vi "Path_Decider.vi"(7 "Second":T3=enum."5", 8 "First":T3=enum."7", 9 "Starting Position":T1) -> (0 "Complete Path Valid?":bool, 1 "Score Second HP Leg":T2={"First Path"="BLANK", "Second Path Needed?"=FALSE, "Second Path"="BLANK"}, 2 "Retrieve Second HP Leg":T2={"First Path"="BLANK", "Second Path Needed?"=FALSE, "Second Path"="BLANK"}, 3 "Score First HP Leg":T2={"First Path"="BLANK", "Second Path Needed?"=FALSE, "Second Path"="BLANK"})   [LabVIEW 2018]
uses:
  Path_Decider.ctl
  pathLeg.ctl
  StartingPosition.ctl
panel:
  in  "Starting Left?":bool
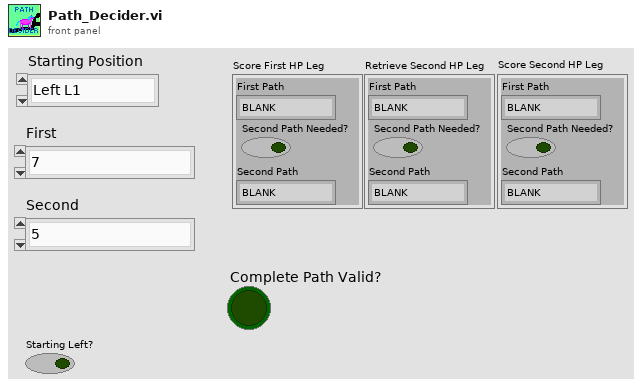
[diagram p1: front panel]
types:
  T1 = typedef "StartingPosition.ctl" = enum16{"Left L1 ", "Middle L1", "Right L1", "Left L2", "Right L2", "Don't Move"}
  T2 = typedef "pathLeg.ctl" = cluster{"First Path":string, "Second Path Needed?":bool, "Second Path":string}
  T3 = typedef "Path_Decider.ctl" = enum16{"1", "2", "3", "4", "5", "6", "7", "8", "Left_Rocket_Front", "Left_Rocket_Rear", "Right_Rocket_Front", "Right_Rocket_Rear"}
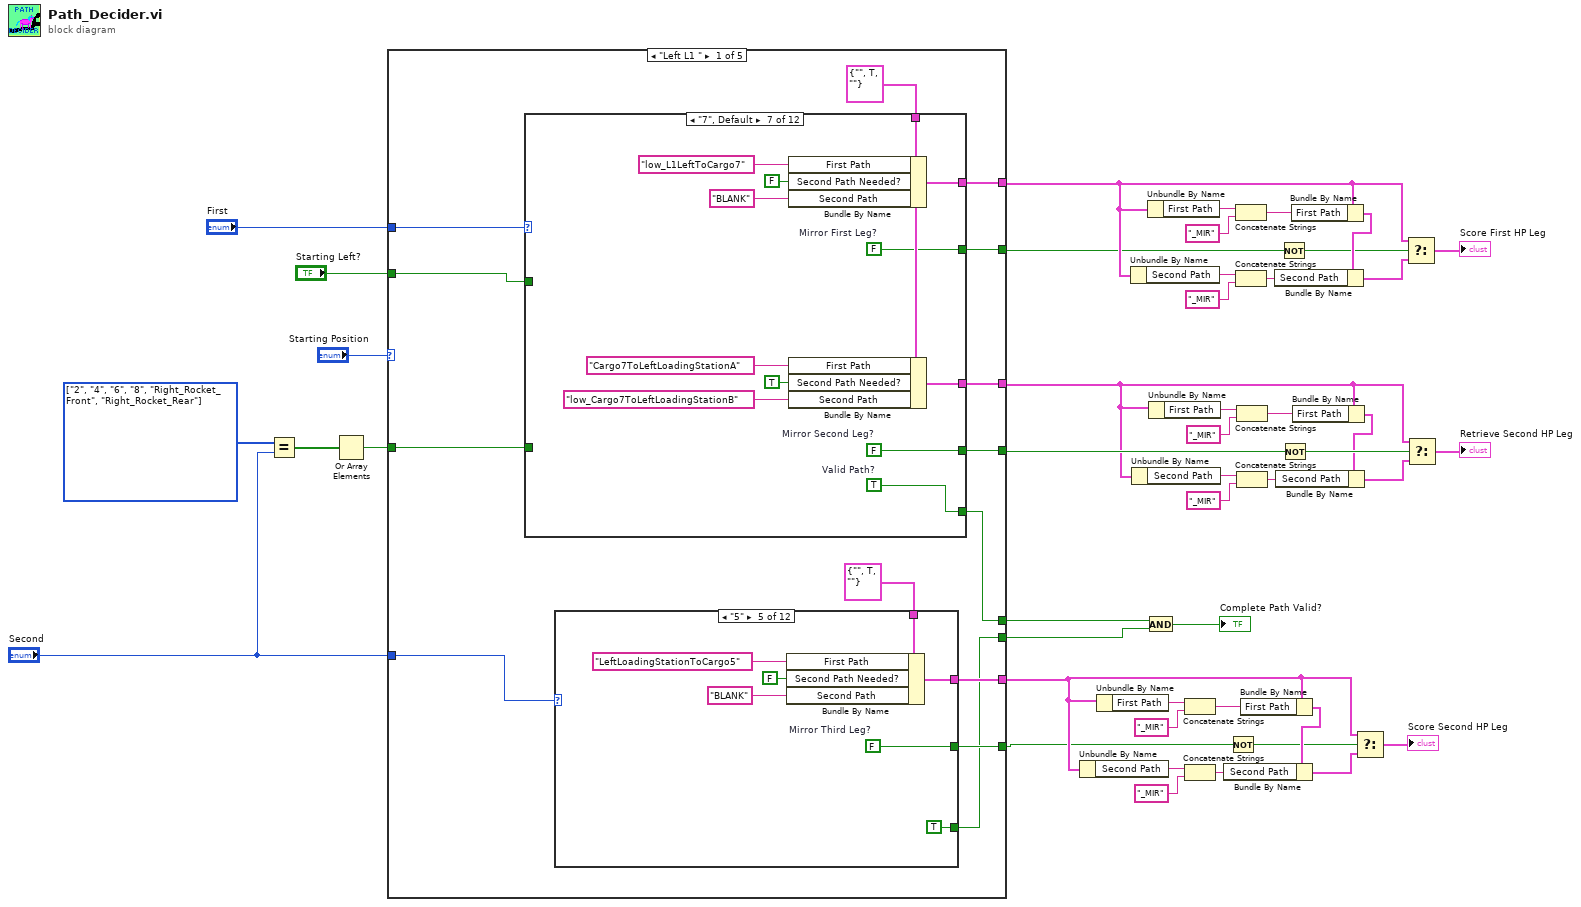
[diagram p0: block diagram]
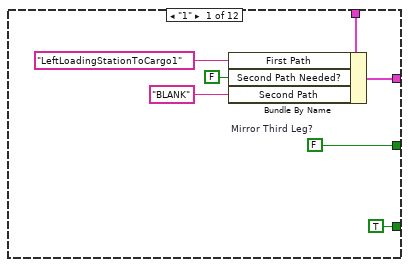
[diagram p2: hidden frame]
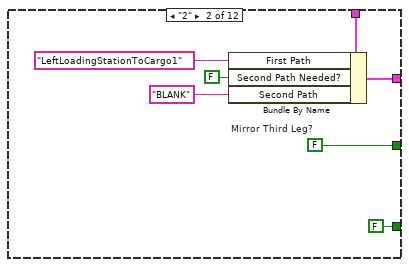
[diagram p3: hidden frame]
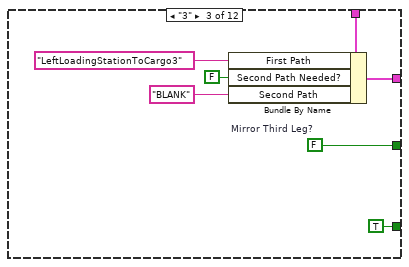
[diagram p4: hidden frame]
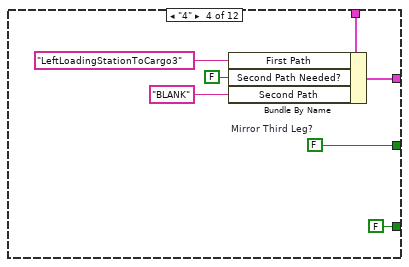
[diagram p5: hidden frame]
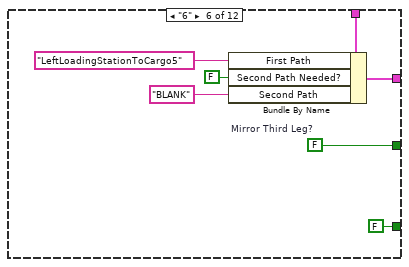
[diagram p6: hidden frame]
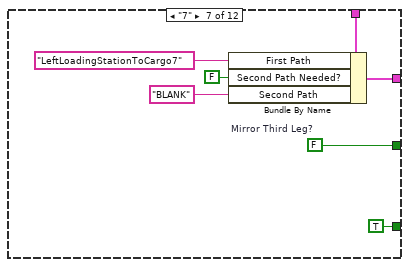
[diagram p7: hidden frame]
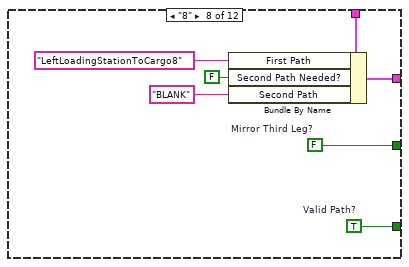
[diagram p8: hidden frame]
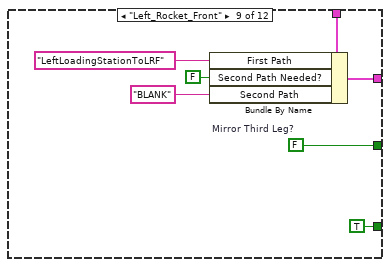
[diagram p9: hidden frame]
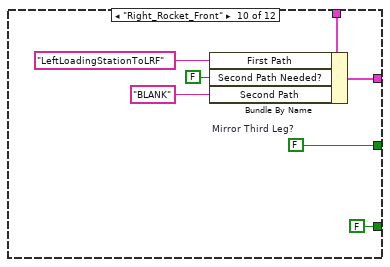
[diagram p10: hidden frame]
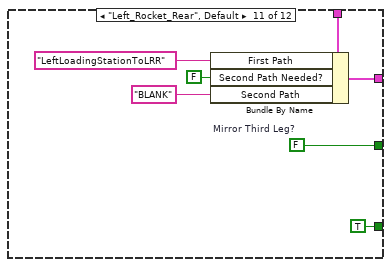
[diagram p11: hidden frame]
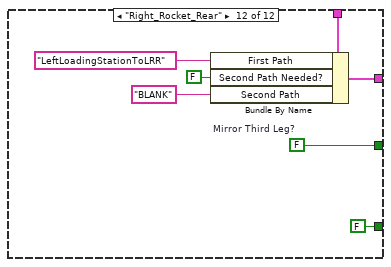
[diagram p12: hidden frame]
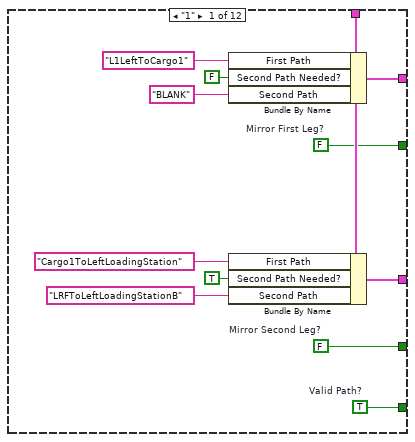
[diagram p13: hidden frame]
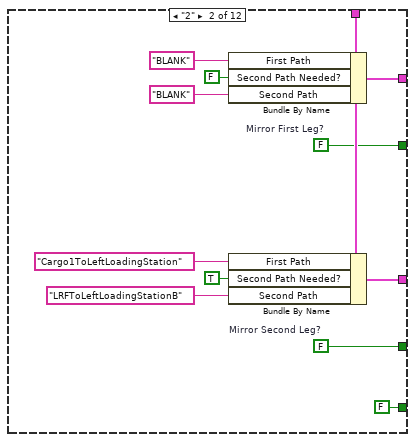
[diagram p14: hidden frame]
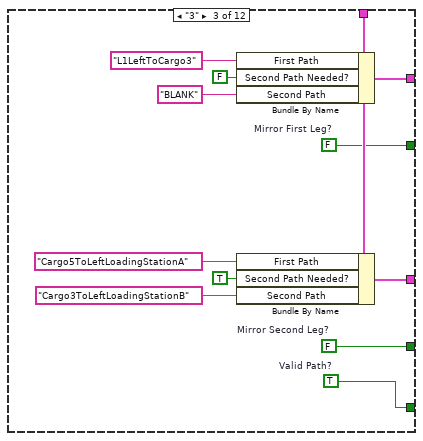
[diagram p15: hidden frame]
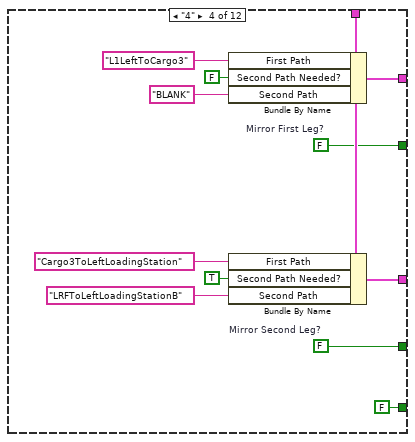
[diagram p16: hidden frame]
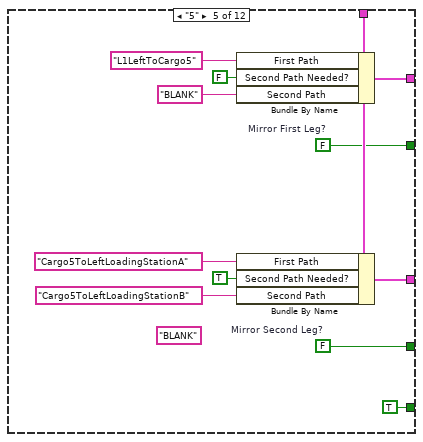
[diagram p17: hidden frame]
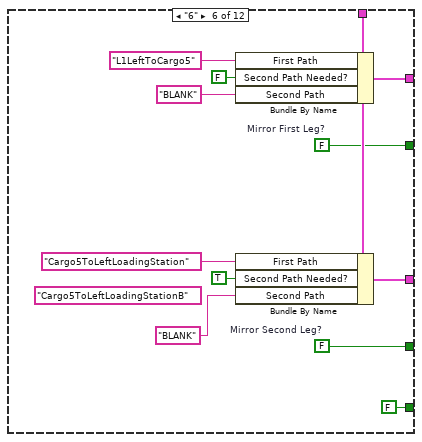
[diagram p18: hidden frame]
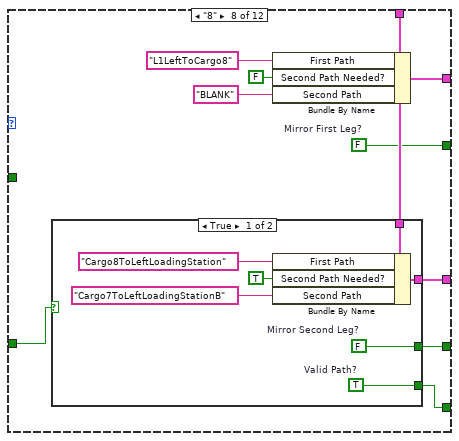
[diagram p19: hidden frame]
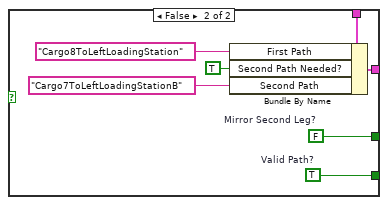
[diagram p20: hidden frame]
diagram:
  w2 = T3[] [enum."2", enum."4", enum."6", enum."8", enum."Right_Rocket_Front", enum."Right_Rocket_Rear"] items=["1", "2", "3", "4", "5", "6", "7", "8", "Left_Rocket_Front", "Left_Rocket_Rear", "Right_Rocket_Front", "Right_Rocket_Rear"] ("array of clusters")
  n1 = Equal?(x=w2, y="Second") -> (x = y?=w4:bool[])
  n2 = Or Array Elements(Boolean array=w4) -> (logical OR=w3:bool)
  n3 = case shown="\"Left L1 \"" "Starting Position" {
    tunnel: [w59 w312 w554 w819 w1060] -> w46
    tunnel: [w58 w311 w553 w818 w1059] -> w45
    tunnel: [w57 w310 w552 w817 w1058] -> w44
    tunnel: [w56 w309 w551 w816 w1057] -> w43
    tunnel: [w54 w307 w549 w814 w1055] -> w42
    tunnel: [w53 w306 w548 w813 w1054] -> w41
    tunnel: "First" -> [w52 w305 w544 w812 w1053]
    tunnel: "Second" -> [w51 w304 w546 w810 w1051]
    tunnel: "Starting Left?" -> [w50 w303 w547 w811 w1052]
    tunnel: [w49 w301 w543 w809 w1050] -> w8
    tunnel: [w48 w302 w545 w808 w1049] -> w7
    tunnel: w3 -> [w47 _ w542 _ _]
    frame "Left L1 " {
      n4 = case shown="\"7\", Default" w52 {
        tunnel: T2 {"First Path"="", "Second Path Needed?"=TRUE, "Second Path"=""} ("pathLeg") -> [w149 w161 w173 w185 w198 w210 w224 w234 w257 w269 w281 w293]
        tunnel: [w156 w168 w180 w192 w204 w216 w228 w238 w264 w276 w288 w300] -> w59
        tunnel: [w148 w160 w172 w184 w197 w209 w223 w233 w256 w268 w280 w292] -> w56
        tunnel: [w147 w159 w171 w183 w196 w208 w222 w232 w255 w267 w279 w291] -> w58
        tunnel: [w146 w158 w170 w182 w195 w207 w221 w231 w254 w266 w278 w290] -> w57
        tunnel: w50 -> [_ _ _ _ _ _ _ _ _ _ _ _]
        tunnel: [w145 FALSE ("Valid Path?") w169 FALSE ("Valid Path?") TRUE ("Valid Path?") FALSE ("Valid Path?") w220 w230 TRUE ("Valid Path?") TRUE ("Valid Path?") FALSE ("Valid Path?") FALSE ("Valid Path?")] -> w49
        tunnel: w47 -> [_ _ _ _ _ _ _ w229 _ _ _ _]
        frame "1" {
          w145 = TRUE  # Valid Path?
          w146 = FALSE  # Mirror Second Leg?
          w147 = FALSE  # Mirror First Leg?
          n5 = Bundle By Name(cluster=w149, "First Path"="L1LeftToCargo1" ("motionProfilePathName"), "Second Path Needed?"=FALSE, "Second Path"="BLANK") -> (w156:T2)
          n6 = Bundle By Name(cluster=w149, "First Path"="Cargo1ToLeftLoadingStation" ("motionProfilePathName"), "Second Path Needed?"=TRUE, "Second Path"="LRFToLeftLoadingStationB") -> (w148:T2)
        }
        frame "2" {
          w158 = FALSE  # Mirror Second Leg?
          w159 = FALSE  # Mirror First Leg?
          n7 = Bundle By Name(cluster=w161, "First Path"="BLANK" ("motionProfilePathName"), "Second Path Needed?"=FALSE, "Second Path"="BLANK") -> (w168:T2)
          n8 = Bundle By Name(cluster=w161, "First Path"="Cargo1ToLeftLoadingStation" ("motionProfilePathName"), "Second Path Needed?"=TRUE, "Second Path"="LRFToLeftLoadingStationB") -> (w160:T2)
        }
        frame "3" {
          w169 = TRUE  # Valid Path?
          w170 = FALSE  # Mirror Second Leg?
          w171 = FALSE  # Mirror First Leg?
          n9 = Bundle By Name(cluster=w173, "First Path"="L1LeftToCargo3" ("motionProfilePathName"), "Second Path Needed?"=FALSE, "Second Path"="BLANK") -> (w180:T2)
          n10 = Bundle By Name(cluster=w173, "First Path"="Cargo5ToLeftLoadingStationA" ("motionProfilePathName"), "Second Path Needed?"=TRUE, "Second Path"="Cargo3ToLeftLoadingStationB") -> (w172:T2)
        }
        frame "4" {
          w182 = FALSE  # Mirror Second Leg?
          w183 = FALSE  # Mirror First Leg?
          n11 = Bundle By Name(cluster=w185, "First Path"="L1LeftToCargo3" ("motionProfilePathName"), "Second Path Needed?"=FALSE, "Second Path"="BLANK") -> (w192:T2)
          n12 = Bundle By Name(cluster=w185, "First Path"="Cargo3ToLeftLoadingStation" ("motionProfilePathName"), "Second Path Needed?"=TRUE, "Second Path"="LRFToLeftLoadingStationB") -> (w184:T2)
        }
        frame "5" {
          (unwired) "BLANK" ("Second Path")
          w195 = FALSE  # Mirror Second Leg?
          w196 = FALSE  # Mirror First Leg?
          n13 = Bundle By Name(cluster=w198, "First Path"="L1LeftToCargo5" ("motionProfilePathName"), "Second Path Needed?"=FALSE, "Second Path"="BLANK") -> (w204:T2)
          n14 = Bundle By Name(cluster=w198, "First Path"="Cargo5ToLeftLoadingStationA" ("motionProfilePathName"), "Second Path Needed?"=TRUE, "Second Path"="Cargo5ToLeftLoadingStationB") -> (w197:T2)
        }
        frame "6" {
          w207 = FALSE  # Mirror Second Leg?
          w208 = FALSE  # Mirror First Leg?
          (unwired) "Cargo5ToLeftLoadingStationB" ("Second Path")
          n15 = Bundle By Name(cluster=w210, "First Path"="L1LeftToCargo5" ("motionProfilePathName"), "Second Path Needed?"=FALSE, "Second Path"="BLANK") -> (w216:T2)
          n16 = Bundle By Name(cluster=w210, "First Path"="Cargo5ToLeftLoadingStation" ("motionProfilePathName"), "Second Path Needed?"=TRUE, "Second Path"="BLANK") -> (w209:T2)
        }
        frame "7", Default {
          w220 = TRUE  # Valid Path?
          w221 = FALSE  # Mirror Second Leg?
          w222 = FALSE  # Mirror First Leg?
          n17 = Bundle By Name(cluster=w224, "First Path"="low_L1LeftToCargo7" ("motionProfilePathName"), "Second Path Needed?"=FALSE, "Second Path"="BLANK") -> (w228:T2)
          n18 = Bundle By Name(cluster=w224, "First Path"="Cargo7ToLeftLoadingStationA" ("motionProfilePathName"), "Second Path Needed?"=TRUE, "Second Path"="low_Cargo7ToLeftLoadingStationB") -> (w223:T2)
        }
        frame "8" {
          w232 = FALSE  # Mirror First Leg?
          n19 = case shown="True" w229 {
            tunnel: w234 -> [w242 w249]
            tunnel: [w241 w248] -> w233
            tunnel: [w240 w247] -> w231
            tunnel: [w239 w246] -> w230
            frame True {
              w239 = TRUE  # Valid Path?
              w240 = FALSE  # Mirror Second Leg?
              n20 = Bundle By Name(cluster=w242, "First Path"="Cargo8ToLeftLoadingStation" ("motionProfilePathName"), "Second Path Needed?"=TRUE, "Second Path"="Cargo7ToLeftLoadingStationB") -> (w241:T2)
            }
            frame False {
              w246 = TRUE  # Valid Path?
              w247 = FALSE  # Mirror Second Leg?
              n21 = Bundle By Name(cluster=w249, "First Path"="Cargo8ToLeftLoadingStation" ("motionProfilePathName"), "Second Path Needed?"=TRUE, "Second Path"="Cargo7ToLeftLoadingStationB") -> (w248:T2)
            }
          }
          n22 = Bundle By Name(cluster=w234, "First Path"="L1LeftToCargo8" ("motionProfilePathName"), "Second Path Needed?"=FALSE, "Second Path"="BLANK") -> (w238:T2)
        }
        frame "Left_Rocket_Front" {
          w254 = FALSE  # Mirror Second Leg?
          w255 = FALSE  # Mirror First Leg?
          n23 = Bundle By Name(cluster=w257, "First Path"="L1LeftToLRF" ("motionProfilePathName"), "Second Path Needed?"=FALSE, "Second Path"="BLANK") -> (w264:T2)
          n24 = Bundle By Name(cluster=w257, "First Path"="LRFToLeftLoadingStationA" ("motionProfilePathName"), "Second Path Needed?"=TRUE, "Second Path"="LRFToLeftLoadingStationB") -> (w256:T2)
        }
        frame "Left_Rocket_Rear" {
          w266 = FALSE  # Mirror Second Leg?
          w267 = FALSE  # Mirror First Leg?
          n25 = Bundle By Name(cluster=w269, "First Path"="L1LeftToLRR" ("motionProfilePathName"), "Second Path Needed?"=FALSE, "Second Path"="BLANK") -> (w276:T2)
          n26 = Bundle By Name(cluster=w269, "First Path"="LRRToLeftLoadingStationA" ("motionProfilePathName"), "Second Path Needed?"=TRUE, "Second Path"="LRRToLeftLoadingStationB") -> (w268:T2)
        }
        frame "Right_Rocket_Rear" {
          w278 = FALSE  # Mirror Second Leg?
          w279 = FALSE  # Mirror First Leg?
          n27 = Bundle By Name(cluster=w281, "First Path"="L1LeftToLRR" ("motionProfilePathName"), "Second Path Needed?"=FALSE, "Second Path"="BLANK") -> (w288:T2)
          n28 = Bundle By Name(cluster=w281, "First Path"="LRRToLeftLoadingStationA" ("motionProfilePathName"), "Second Path Needed?"=TRUE, "Second Path"="LRRToLeftLoadingStationB") -> (w280:T2)
        }
        frame "Right_Rocket_Front" {
          w290 = FALSE  # Mirror Second Leg?
          w291 = FALSE  # Mirror First Leg?
          n29 = Bundle By Name(cluster=w293, "First Path"="L1LeftToLRR" ("motionProfilePathName"), "Second Path Needed?"=FALSE, "Second Path"="BLANK") -> (w300:T2)
          n30 = Bundle By Name(cluster=w293, "First Path"="LRRToLeftLoadingStationA" ("motionProfilePathName"), "Second Path Needed?"=TRUE, "Second Path"="LRRToLeftLoadingStationB") -> (w292:T2)
        }
      }
      n31 = case shown="\"5\"" w51 {
        tunnel: T2 {"First Path"="", "Second Path Needed?"=TRUE, "Second Path"=""} ("pathLeg") -> [w64 w71 w78 w85 w92 w99 w106 w113 w120 w127 w134 w141]
        tunnel: [w63 w70 w77 w84 w91 w98 w105 w112 w119 w126 w133 w140] -> w54
        tunnel: [w62 w69 w76 w83 w90 w97 w104 w111 w118 w125 w132 w139] -> w53
        tunnel: [TRUE ("Valid Path?") FALSE ("Valid Path?") TRUE ("Valid Path?") FALSE ("Valid Path?") TRUE ("Valid Path?") FALSE ("Valid Path?") TRUE ("Valid Path?") w110 TRUE ("Valid Path?") FALSE ("Valid Path?") TRUE ("Valid Path?") FALSE ("Valid Path?")] -> w48
        frame "1" {
          w62 = FALSE  # Mirror Third Leg?
          n32 = Bundle By Name(cluster=w64, "First Path"="LeftLoadingStationToCargo1" ("motionProfilePathName"), "Second Path Needed?"=FALSE, "Second Path"="BLANK") -> (w63:T2)
        }
        frame "2" {
          w69 = FALSE  # Mirror Third Leg?
          n33 = Bundle By Name(cluster=w71, "First Path"="LeftLoadingStationToCargo1" ("motionProfilePathName"), "Second Path Needed?"=FALSE, "Second Path"="BLANK") -> (w70:T2)
        }
        frame "3" {
          w76 = FALSE  # Mirror Third Leg?
          n34 = Bundle By Name(cluster=w78, "First Path"="LeftLoadingStationToCargo3" ("motionProfilePathName"), "Second Path Needed?"=FALSE, "Second Path"="BLANK") -> (w77:T2)
        }
        frame "4" {
          w83 = FALSE  # Mirror Third Leg?
          n35 = Bundle By Name(cluster=w85, "First Path"="LeftLoadingStationToCargo3" ("motionProfilePathName"), "Second Path Needed?"=FALSE, "Second Path"="BLANK") -> (w84:T2)
        }
        frame "5" {
          w90 = FALSE  # Mirror Third Leg?
          n36 = Bundle By Name(cluster=w92, "First Path"="LeftLoadingStationToCargo5" ("motionProfilePathName"), "Second Path Needed?"=FALSE, "Second Path"="BLANK") -> (w91:T2)
        }
        frame "6" {
          w97 = FALSE  # Mirror Third Leg?
          n37 = Bundle By Name(cluster=w99, "First Path"="LeftLoadingStationToCargo5" ("motionProfilePathName"), "Second Path Needed?"=FALSE, "Second Path"="BLANK") -> (w98:T2)
        }
        frame "7" {
          w104 = FALSE  # Mirror Third Leg?
          n38 = Bundle By Name(cluster=w106, "First Path"="LeftLoadingStationToCargo7" ("motionProfilePathName"), "Second Path Needed?"=FALSE, "Second Path"="BLANK") -> (w105:T2)
        }
        frame "8" {
          w110 = TRUE  # Valid Path?
          w111 = FALSE  # Mirror Third Leg?
          n39 = Bundle By Name(cluster=w113, "First Path"="LeftLoadingStationToCargo8" ("motionProfilePathName"), "Second Path Needed?"=FALSE, "Second Path"="BLANK") -> (w112:T2)
        }
        frame "Left_Rocket_Front" {
          w118 = FALSE  # Mirror Third Leg?
          n40 = Bundle By Name(cluster=w120, "First Path"="LeftLoadingStationToLRF" ("motionProfilePathName"), "Second Path Needed?"=FALSE, "Second Path"="BLANK") -> (w119:T2)
        }
        frame "Right_Rocket_Front" {
          w125 = FALSE  # Mirror Third Leg?
          n41 = Bundle By Name(cluster=w127, "First Path"="LeftLoadingStationToLRF" ("motionProfilePathName"), "Second Path Needed?"=FALSE, "Second Path"="BLANK") -> (w126:T2)
        }
        frame "Left_Rocket_Rear", Default {
          w132 = FALSE  # Mirror Third Leg?
          n42 = Bundle By Name(cluster=w134, "First Path"="LeftLoadingStationToLRR" ("motionProfilePathName"), "Second Path Needed?"=FALSE, "Second Path"="BLANK") -> (w133:T2)
        }
        frame "Right_Rocket_Rear" {
          w139 = FALSE  # Mirror Third Leg?
          n43 = Bundle By Name(cluster=w141, "First Path"="LeftLoadingStationToLRR" ("motionProfilePathName"), "Second Path Needed?"=FALSE, "Second Path"="BLANK") -> (w140:T2)
        }
      }
    }
    frame "Middle L1", Default {
      n44 = case shown="\"5\"" w304 {
        tunnel: T2 {"First Path"="", "Second Path Needed?"=TRUE, "Second Path"=""} ("pathLeg") -> [w317 w324 w331 w338 w345 w352 w359 w366 w373 w380 w387 w394]
        tunnel: [w316 w323 w330 w337 w344 w351 w358 w365 w372 w379 w386 w393] -> w307
        tunnel: [w315 w322 w329 w336 w343 w350 w357 w364 w371 w378 w385 w392] -> w306
        tunnel: [w314 w321 w328 w335 w342 w349 w356 w363 w370 w377 w384 w391] -> w302
        frame "1" {
          w314 = FALSE  # Valid Path?
          w315 = FALSE  # Mirror Third Leg?
          n45 = Bundle By Name(cluster=w317, "First Path"="LeftLoadingStationToCargo1" ("motionProfilePathName"), "Second Path Needed?"=FALSE, "Second Path"="BLANK") -> (w316:T2)
        }
        frame "2" {
          w321 = FALSE  # Valid Path?
          w322 = FALSE  # Mirror Third Leg?
          n46 = Bundle By Name(cluster=w324, "First Path"="LeftLoadingStationToCargo1" ("motionProfilePathName"), "Second Path Needed?"=FALSE, "Second Path"="BLANK") -> (w323:T2)
        }
        frame "3" {
          w328 = FALSE  # Valid Path?
          w329 = FALSE  # Mirror Third Leg?
          n47 = Bundle By Name(cluster=w331, "First Path"="LeftLoadingStationToCargo3" ("motionProfilePathName"), "Second Path Needed?"=FALSE, "Second Path"="BLANK") -> (w330:T2)
        }
        frame "4" {
          w335 = FALSE  # Valid Path?
          w336 = FALSE  # Mirror Third Leg?
          n48 = Bundle By Name(cluster=w338, "First Path"="LeftLoadingStationToCargo3" ("motionProfilePathName"), "Second Path Needed?"=FALSE, "Second Path"="BLANK") -> (w337:T2)
        }
        frame "5" {
          w342 = TRUE  # Valid Path?
          w343 = TRUE  # Mirror Third Leg?
          n49 = Bundle By Name(cluster=w345, "First Path"="RightLoadingStationToCargo6" ("motionProfilePathName"), "Second Path Needed?"=FALSE, "Second Path"="BLANK") -> (w344:T2)
        }
        frame "6" {
          w349 = TRUE  # Valid Path?
          w350 = FALSE  # Mirror Third Leg?
          n50 = Bundle By Name(cluster=w352, "First Path"="RightLoadingStationToCargo6" ("motionProfilePathName"), "Second Path Needed?"=FALSE, "Second Path"="BLANK") -> (w351:T2)
        }
        frame "7" {
          w356 = FALSE  # Valid Path?
          w357 = FALSE  # Mirror Third Leg?
          n51 = Bundle By Name(cluster=w359, "First Path"="LeftLoadingStationToCargo7" ("motionProfilePathName"), "Second Path Needed?"=FALSE, "Second Path"="BLANK") -> (w358:T2)
        }
        frame "8" {
          w363 = FALSE  # Valid Path?
          w364 = FALSE  # Mirror Third Leg?
          n52 = Bundle By Name(cluster=w366, "First Path"="LeftLoadingStationToCargo8" ("motionProfilePathName"), "Second Path Needed?"=FALSE, "Second Path"="BLANK") -> (w365:T2)
        }
        frame "Left_Rocket_Front" {
          w370 = TRUE  # Valid Path?
          w371 = FALSE  # Mirror Third Leg?
          n53 = Bundle By Name(cluster=w373, "First Path"="LeftLoadingStationToLRF" ("motionProfilePathName"), "Second Path Needed?"=FALSE, "Second Path"="BLANK") -> (w372:T2)
        }
        frame "Right_Rocket_Front" {
          w377 = TRUE  # Valid Path?
          w378 = FALSE  # Mirror Third Leg?
          n54 = Bundle By Name(cluster=w380, "First Path"="LeftLoadingStationToLRF" ("motionProfilePathName"), "Second Path Needed?"=FALSE, "Second Path"="BLANK") -> (w379:T2)
        }
        frame "Left_Rocket_Rear", Default {
          w384 = TRUE  # Valid Path?
          w385 = FALSE  # Mirror Third Leg?
          n55 = Bundle By Name(cluster=w387, "First Path"="LeftLoadingStationToLRR" ("motionProfilePathName"), "Second Path Needed?"=FALSE, "Second Path"="BLANK") -> (w386:T2)
        }
        frame "Right_Rocket_Rear" {
          w391 = TRUE  # Valid Path?
          w392 = FALSE  # Mirror Third Leg?
          n56 = Bundle By Name(cluster=w394, "First Path"="LeftLoadingStationToLRR" ("motionProfilePathName"), "Second Path Needed?"=FALSE, "Second Path"="BLANK") -> (w393:T2)
        }
      }
      n57 = case shown="\"8\"" w305 {
        tunnel: w303 -> [_ _ _ _ _ _ _ _ _ _ _ _]
        tunnel: T2 {"First Path"="", "Second Path Needed?"=TRUE, "Second Path"=""} ("pathLeg") -> [w402 w414 w426 w438 w451 w463 w474 w486 w498 w510 w522 w534]
        tunnel: [w409 w421 w433 w445 w457 w469 w481 w493 w505 w517 w529 w541] -> w312
        tunnel: [w401 w413 w425 w437 w450 w462 w473 w485 w497 w509 w521 w533] -> w309
        tunnel: [w400 w412 w424 w436 w449 w461 w472 w484 w496 w508 w520 w532] -> w311
        tunnel: [w399 w411 w423 w435 w448 w460 w471 w483 w495 w507 w519 w531] -> w310
        tunnel: [w398 w410 w422 w434 w446 w458 w470 w482 w494 w506 w518 w530] -> w301
        frame "1" {
          w398 = FALSE  # Valid Path?
          w399 = FALSE  # Mirror Second Leg?
          w400 = FALSE  # Mirror First Leg?
          n58 = Bundle By Name(cluster=w402, "First Path"="BLANK" ("motionProfilePathName"), "Second Path Needed?"=FALSE, "Second Path"="BLANK") -> (w409:T2)
          n59 = Bundle By Name(cluster=w402, "First Path"="Cargo1ToLeftLoadingStation" ("motionProfilePathName"), "Second Path Needed?"=TRUE, "Second Path"="LRFToLeftLoadingStationB") -> (w401:T2)
        }
        frame "2" {
          w410 = FALSE  # Valid Path?
          w411 = FALSE  # Mirror Second Leg?
          w412 = FALSE  # Mirror First Leg?
          n60 = Bundle By Name(cluster=w414, "First Path"="BLANK" ("motionProfilePathName"), "Second Path Needed?"=FALSE, "Second Path"="BLANK") -> (w421:T2)
          n61 = Bundle By Name(cluster=w414, "First Path"="Cargo1ToLeftLoadingStation" ("motionProfilePathName"), "Second Path Needed?"=TRUE, "Second Path"="LRFToLeftLoadingStationB") -> (w413:T2)
        }
        frame "3" {
          w422 = FALSE  # Valid Path?
          w423 = FALSE  # Mirror Second Leg?
          w424 = FALSE  # Mirror First Leg?
          n62 = Bundle By Name(cluster=w426, "First Path"="BLANK" ("motionProfilePathName"), "Second Path Needed?"=FALSE, "Second Path"="BLANK") -> (w433:T2)
          n63 = Bundle By Name(cluster=w426, "First Path"="Cargo3ToLeftLoadingStation" ("motionProfilePathName"), "Second Path Needed?"=TRUE, "Second Path"="LRFToLeftLoadingStationB") -> (w425:T2)
        }
        frame "4" {
          w434 = FALSE  # Valid Path?
          w435 = FALSE  # Mirror Second Leg?
          w436 = FALSE  # Mirror First Leg?
          n64 = Bundle By Name(cluster=w438, "First Path"="BLANK" ("motionProfilePathName"), "Second Path Needed?"=FALSE, "Second Path"="BLANK") -> (w445:T2)
          n65 = Bundle By Name(cluster=w438, "First Path"="Cargo3ToLeftLoadingStation" ("motionProfilePathName"), "Second Path Needed?"=TRUE, "Second Path"="LRFToLeftLoadingStationB") -> (w437:T2)
        }
        frame "5" {
          w446 = FALSE  # Valid Path?
          w448 = FALSE  # Mirror Second Leg?
          w449 = FALSE  # Mirror First Leg?
          (unwired) "Cargo5ToLeftLoadingStationB" ("Second Path")
          n66 = Bundle By Name(cluster=w451, "First Path"="BLANK" ("motionProfilePathName"), "Second Path Needed?"=FALSE, "Second Path"="BLANK") -> (w457:T2)
          n67 = Bundle By Name(cluster=w451, "First Path"="Cargo5ToLeftLoadingStation" ("motionProfilePathName"), "Second Path Needed?"=TRUE, "Second Path"="BLANK") -> (w450:T2)
        }
        frame "6" {
          w458 = FALSE  # Valid Path?
          w460 = FALSE  # Mirror Second Leg?
          w461 = FALSE  # Mirror First Leg?
          (unwired) "Cargo5ToLeftLoadingStationB" ("Second Path")
          n68 = Bundle By Name(cluster=w463, "First Path"="BLANK" ("motionProfilePathName"), "Second Path Needed?"=FALSE, "Second Path"="BLANK") -> (w469:T2)
          n69 = Bundle By Name(cluster=w463, "First Path"="Cargo5ToLeftLoadingStation" ("motionProfilePathName"), "Second Path Needed?"=TRUE, "Second Path"="BLANK") -> (w462:T2)
        }
        frame "7", Default {
          w470 = TRUE  # Valid Path?
          w471 = FALSE  # Mirror Second Leg?
          w472 = FALSE  # Mirror First Leg?
          n70 = Bundle By Name(cluster=w474, "First Path"="low_L1MiddleToCargo7" ("motionProfilePathName"), "Second Path Needed?"=FALSE, "Second Path"="BLANK") -> (w481:T2)
          n71 = Bundle By Name(cluster=w474, "First Path"="Cargo7ToLeftLoadingStationA" ("motionProfilePathName"), "Second Path Needed?"=TRUE, "Second Path"="low_Cargo7ToLeftLoadingStationB") -> (w473:T2)
        }
        frame "8" {
          w482 = TRUE  # Valid Path?
          w483 = FALSE  # Mirror Second Leg?
          w484 = TRUE  # Mirror First Leg?
          n72 = Bundle By Name(cluster=w486, "First Path"="low_L1MiddleToCargo7" ("motionProfilePathName"), "Second Path Needed?"=FALSE, "Second Path"="BLANK") -> (w493:T2)
          n73 = Bundle By Name(cluster=w486, "First Path"="Cargo8ToRightLoadingStationA" ("motionProfilePathName"), "Second Path Needed?"=TRUE, "Second Path"="low_Cargo8ToRightLoadingStationB") -> (w485:T2)
        }
        frame "Left_Rocket_Front" {
          w494 = FALSE  # Valid Path?
          w495 = FALSE  # Mirror Second Leg?
          w496 = FALSE  # Mirror First Leg?
          n74 = Bundle By Name(cluster=w498, "First Path"="BLANK" ("motionProfilePathName"), "Second Path Needed?"=FALSE, "Second Path"="BLANK") -> (w505:T2)
          n75 = Bundle By Name(cluster=w498, "First Path"="LRFToLeftLoadingStationA" ("motionProfilePathName"), "Second Path Needed?"=TRUE, "Second Path"="LRFToLeftLoadingStationB") -> (w497:T2)
        }
        frame "Left_Rocket_Rear" {
          w506 = FALSE  # Valid Path?
          w507 = FALSE  # Mirror Second Leg?
          w508 = FALSE  # Mirror First Leg?
          n76 = Bundle By Name(cluster=w510, "First Path"="BLANK" ("motionProfilePathName"), "Second Path Needed?"=FALSE, "Second Path"="BLANK") -> (w517:T2)
          n77 = Bundle By Name(cluster=w510, "First Path"="LRRToLeftLoadingStationA" ("motionProfilePathName"), "Second Path Needed?"=TRUE, "Second Path"="LRRToLeftLoadingStationB") -> (w509:T2)
        }
        frame "Right_Rocket_Rear" {
          w518 = FALSE  # Valid Path?
          w519 = FALSE  # Mirror Second Leg?
          w520 = FALSE  # Mirror First Leg?
          n78 = Bundle By Name(cluster=w522, "First Path"="BLANK" ("motionProfilePathName"), "Second Path Needed?"=FALSE, "Second Path"="BLANK") -> (w529:T2)
          n79 = Bundle By Name(cluster=w522, "First Path"="LRRToLeftLoadingStationA" ("motionProfilePathName"), "Second Path Needed?"=TRUE, "Second Path"="LRRToLeftLoadingStationB") -> (w521:T2)
        }
        frame "Right_Rocket_Front" {
          w530 = FALSE  # Valid Path?
          w531 = FALSE  # Mirror Second Leg?
          w532 = FALSE  # Mirror First Leg?
          n80 = Bundle By Name(cluster=w534, "First Path"="BLANK" ("motionProfilePathName"), "Second Path Needed?"=FALSE, "Second Path"="BLANK") -> (w541:T2)
          n81 = Bundle By Name(cluster=w534, "First Path"="LRRToLeftLoadingStationA" ("motionProfilePathName"), "Second Path Needed?"=TRUE, "Second Path"="LRRToLeftLoadingStationB") -> (w533:T2)
        }
      }
    }
    frame "Right L1" {
      n82 = case shown="\"4\"" w546 {
        tunnel: T2 {"First Path"="", "Second Path Needed?"=TRUE, "Second Path"=""} ("pathLeg") -> [w559 w566 w573 w580 w587 w594 w601 w608 w615 w622 w629 w636]
        tunnel: [w558 w565 w572 w579 w586 w593 w600 w607 w614 w621 w628 w635] -> w549
        tunnel: [w557 w564 w571 w578 w585 w592 w599 w606 w613 w620 w627 w634] -> w548
        tunnel: [FALSE ("Valid Path?") TRUE ("Valid Path?") FALSE ("Valid Path?") w577 FALSE ("Valid Path?") TRUE ("Valid Path?") TRUE ("Valid Path?") TRUE ("Valid Path?") FALSE ("Valid Path?") TRUE ("Valid Path?") FALSE ("Valid Path?") w633] -> w545
        frame "1" {
          w557 = FALSE  # Mirror Third Leg?
          n83 = Bundle By Name(cluster=w559, "First Path"="LeftLoadingStationToCargo1" ("motionProfilePathName"), "Second Path Needed?"=FALSE, "Second Path"="BLANK") -> (w558:T2)
        }
        frame "2" {
          w564 = TRUE  # Mirror Third Leg?
          n84 = Bundle By Name(cluster=w566, "First Path"="LeftLoadingStationToCargo1" ("motionProfilePathName"), "Second Path Needed?"=FALSE, "Second Path"="BLANK") -> (w565:T2)
        }
        frame "3" {
          w571 = FALSE  # Mirror Third Leg?
          n85 = Bundle By Name(cluster=w573, "First Path"="LeftLoadingStationToCargo3" ("motionProfilePathName"), "Second Path Needed?"=FALSE, "Second Path"="BLANK") -> (w572:T2)
        }
        frame "4" {
          w577 = TRUE  # Valid Path?
          w578 = TRUE  # Mirror Third Leg?
          n86 = Bundle By Name(cluster=w580, "First Path"="LeftLoadingStationToCargo3" ("motionProfilePathName"), "Second Path Needed?"=FALSE, "Second Path"="BLANK") -> (w579:T2)
        }
        frame "5" {
          w585 = FALSE  # Mirror Third Leg?
          n87 = Bundle By Name(cluster=w587, "First Path"="LeftLoadingStationToCargo5" ("motionProfilePathName"), "Second Path Needed?"=FALSE, "Second Path"="BLANK") -> (w586:T2)
        }
        frame "6" {
          w592 = FALSE  # Mirror Third Leg?
          n88 = Bundle By Name(cluster=w594, "First Path"="RightLoadingStationToCargo6" ("motionProfilePathName"), "Second Path Needed?"=FALSE, "Second Path"="BLANK") -> (w593:T2)
        }
        frame "7" {
          w599 = TRUE  # Mirror Third Leg?
          n89 = Bundle By Name(cluster=w601, "First Path"="LeftLoadingStationToCargo8" ("motionProfilePathName"), "Second Path Needed?"=FALSE, "Second Path"="BLANK") -> (w600:T2)
        }
        frame "8" {
          w606 = TRUE  # Mirror Third Leg?
          n90 = Bundle By Name(cluster=w608, "First Path"="LeftLoadingStationToCargo7" ("motionProfilePathName"), "Second Path Needed?"=FALSE, "Second Path"="BLANK") -> (w607:T2)
        }
        frame "Left_Rocket_Front" {
          w613 = FALSE  # Mirror Third Leg?
          n91 = Bundle By Name(cluster=w615, "First Path"="LeftLoadingStationToLRF" ("motionProfilePathName"), "Second Path Needed?"=FALSE, "Second Path"="BLANK") -> (w614:T2)
        }
        frame "Right_Rocket_Front" {
          w620 = TRUE  # Mirror Third Leg?
          n92 = Bundle By Name(cluster=w622, "First Path"="LeftLoadingStationToLRF" ("motionProfilePathName"), "Second Path Needed?"=FALSE, "Second Path"="BLANK") -> (w621:T2)
        }
        frame "Left_Rocket_Rear", Default {
          w627 = FALSE  # Mirror Third Leg?
          n93 = Bundle By Name(cluster=w629, "First Path"="LeftLoadingStationToLRR" ("motionProfilePathName"), "Second Path Needed?"=FALSE, "Second Path"="BLANK") -> (w628:T2)
        }
        frame "Right_Rocket_Rear" {
          w633 = TRUE  # Valid Path?
          w634 = TRUE  # Mirror Third Leg?
          n94 = Bundle By Name(cluster=w636, "First Path"="LeftLoadingStationToLRR" ("motionProfilePathName"), "Second Path Needed?"=FALSE, "Second Path"="BLANK") -> (w635:T2)
        }
      }
      n95 = case shown="\"5\"" w544 {
        tunnel: T2 {"First Path"="", "Second Path Needed?"=TRUE, "Second Path"=""} ("pathLeg") -> [w644 w656 w668 w680 w693 w705 w717 w741 w764 w776 w788 w800]
        tunnel: [w651 w663 w675 w687 w699 w711 w721 w745 w771 w783 w795 w807] -> w554
        tunnel: [w643 w655 w667 w679 w692 w704 w716 w740 w763 w775 w787 w799] -> w551
        tunnel: [w642 w654 w666 w678 w691 w703 w715 w739 w762 w774 w786 w798] -> w553
        tunnel: [w641 w653 w665 w677 w690 w702 w714 w738 w761 w773 w785 w797] -> w552
        tunnel: w547 -> [_ _ _ _ _ _ _ _ _ _ _ _]
        tunnel: [w640 TRUE ("Valid Path?") FALSE ("Valid Path?") TRUE ("Valid Path?") FALSE ("Valid Path?") TRUE ("Valid Path?") w713 w737 FALSE ("Valid Path?") TRUE ("Valid Path?") FALSE ("Valid Path?") TRUE ("Valid Path?")] -> w543
        tunnel: w542 -> [_ _ _ _ _ _ w712 w736 _ _ _ _]
        frame "1" {
          w640 = FALSE  # Valid Path?
          w641 = FALSE  # Mirror Second Leg?
          w642 = FALSE  # Mirror First Leg?
          n96 = Bundle By Name(cluster=w644, "First Path"="L1LeftToCargo1" ("motionProfilePathName"), "Second Path Needed?"=FALSE, "Second Path"="BLANK") -> (w651:T2)
          n97 = Bundle By Name(cluster=w644, "First Path"="Cargo1ToLeftLoadingStation" ("motionProfilePathName"), "Second Path Needed?"=TRUE, "Second Path"="LRFToLeftLoadingStationB") -> (w643:T2)
        }
        frame "2" {
          w653 = TRUE  # Mirror Second Leg?
          w654 = TRUE  # Mirror First Leg?
          n98 = Bundle By Name(cluster=w656, "First Path"="L1LeftToCargo1" ("motionProfilePathName"), "Second Path Needed?"=FALSE, "Second Path"="BLANK") -> (w663:T2)
          n99 = Bundle By Name(cluster=w656, "First Path"="Cargo1ToLeftLoadingStation" ("motionProfilePathName"), "Second Path Needed?"=TRUE, "Second Path"="LRFToLeftLoadingStationB") -> (w655:T2)
        }
        frame "3" {
          w665 = FALSE  # Mirror Second Leg?
          w666 = FALSE  # Mirror First Leg?
          n100 = Bundle By Name(cluster=w668, "First Path"="L1LeftToCargo3" ("motionProfilePathName"), "Second Path Needed?"=FALSE, "Second Path"="BLANK") -> (w675:T2)
          n101 = Bundle By Name(cluster=w668, "First Path"="Cargo3ToLeftLoadingStation" ("motionProfilePathName"), "Second Path Needed?"=TRUE, "Second Path"="LRFToLeftLoadingStationB") -> (w667:T2)
        }
        frame "4" {
          w677 = TRUE  # Mirror Second Leg?
          w678 = TRUE  # Mirror First Leg?
          n102 = Bundle By Name(cluster=w680, "First Path"="L1LeftToCargo3" ("motionProfilePathName"), "Second Path Needed?"=FALSE, "Second Path"="BLANK") -> (w687:T2)
          n103 = Bundle By Name(cluster=w680, "First Path"="Cargo3ToLeftLoadingStation" ("motionProfilePathName"), "Second Path Needed?"=TRUE, "Second Path"="LRFToLeftLoadingStationB") -> (w679:T2)
        }
        frame "5" {
          w690 = FALSE  # Mirror Second Leg?
          w691 = FALSE  # Mirror First Leg?
          (unwired) "Cargo5ToLeftLoadingStationB" ("Second Path")
          n104 = Bundle By Name(cluster=w693, "First Path"="L1LeftToCargo5" ("motionProfilePathName"), "Second Path Needed?"=FALSE, "Second Path"="BLANK") -> (w699:T2)
          n105 = Bundle By Name(cluster=w693, "First Path"="Cargo5ToLeftLoadingStation" ("motionProfilePathName"), "Second Path Needed?"=TRUE, "Second Path"="BLANK") -> (w692:T2)
        }
        frame "6" {
          (unwired) "BLANK" ("Second Path")
          w702 = TRUE  # Mirror Second Leg?
          w703 = FALSE  # Mirror First Leg?
          n106 = Bundle By Name(cluster=w705, "First Path"="L1RightToCargo6" ("motionProfilePathName"), "Second Path Needed?"=FALSE, "Second Path"="BLANK") -> (w711:T2)
          n107 = Bundle By Name(cluster=w705, "First Path"="Cargo5ToLeftLoadingStationA" ("motionProfilePathName"), "Second Path Needed?"=TRUE, "Second Path"="Cargo5ToLeftLoadingStationB") -> (w704:T2)
        }
        frame "7", Default {
          w715 = TRUE  # Mirror First Leg?
          n108 = case shown="False" w712 {
            tunnel: w717 -> [w725 w732]
            tunnel: [w724 w731] -> w716
            tunnel: [w723 w730] -> w714
            tunnel: [TRUE ("Valid Path?") TRUE ("Valid Path?")] -> w713
            frame True {
              w723 = TRUE  # Mirror Second Leg?
              n109 = Bundle By Name(cluster=w725, "First Path"="Cargo8ToLeftLoadingStationA" ("motionProfilePathName"), "Second Path Needed?"=TRUE, "Second Path"="Cargo8ToLeftLoadingStationB") -> (w724:T2)
            }
            frame False {
              w730 = TRUE  # Mirror Second Leg?
              n110 = Bundle By Name(cluster=w732, "First Path"="Cargo8ToLeftLoadingStationA" ("motionProfilePathName"), "Second Path Needed?"=TRUE, "Second Path"="Cargo8ToLeftLoadingStationB") -> (w731:T2)
            }
          }
          n111 = Bundle By Name(cluster=w717, "First Path"="L1LeftToCargo8" ("motionProfilePathName"), "Second Path Needed?"=FALSE, "Second Path"="BLANK") -> (w721:T2)
        }
        frame "8" {
          w739 = TRUE  # Mirror First Leg?
          n112 = case shown="True" w736 {
            tunnel: w741 -> [w749 w756]
            tunnel: [w748 w755] -> w740
            tunnel: [w747 w754] -> w738
            tunnel: [w746 w753] -> w737
            frame True {
              w746 = TRUE  # Valid Path?
              w747 = FALSE  # Mirror Second Leg?
              n113 = Bundle By Name(cluster=w749, "First Path"="Cargo8ToRightLoadingStationA" ("motionProfilePathName"), "Second Path Needed?"=TRUE, "Second Path"="low_Cargo8ToRightLoadingStationB") -> (w748:T2)
            }
            frame False {
              w753 = TRUE  # Valid Path?
              w754 = TRUE  # Mirror Second Leg?
              n114 = Bundle By Name(cluster=w756, "First Path"="Cargo8ToRightLoadingStationA" ("motionProfilePathName"), "Second Path Needed?"=TRUE, "Second Path"="Cargo7ToLeftLoadingStationB") -> (w755:T2)
            }
          }
          n115 = Bundle By Name(cluster=w741, "First Path"="low_L1LeftToCargo7" ("motionProfilePathName"), "Second Path Needed?"=FALSE, "Second Path"="BLANK") -> (w745:T2)
        }
        frame "Left_Rocket_Front" {
          w761 = FALSE  # Mirror Second Leg?
          w762 = FALSE  # Mirror First Leg?
          n116 = Bundle By Name(cluster=w764, "First Path"="L1LeftToLRF" ("motionProfilePathName"), "Second Path Needed?"=FALSE, "Second Path"="BLANK") -> (w771:T2)
          n117 = Bundle By Name(cluster=w764, "First Path"="LRFToLeftLoadingStationA" ("motionProfilePathName"), "Second Path Needed?"=TRUE, "Second Path"="LRFToLeftLoadingStationB") -> (w763:T2)
        }
        frame "Right_Rocket_Front" {
          w773 = TRUE  # Mirror Second Leg?
          w774 = TRUE  # Mirror First Leg?
          n118 = Bundle By Name(cluster=w776, "First Path"="L1LeftToLRF" ("motionProfilePathName"), "Second Path Needed?"=FALSE, "Second Path"="BLANK") -> (w783:T2)
          n119 = Bundle By Name(cluster=w776, "First Path"="LRFToLeftLoadingStationA" ("motionProfilePathName"), "Second Path Needed?"=TRUE, "Second Path"="LRFToLeftLoadingStationB") -> (w775:T2)
        }
        frame "Left_Rocket_Rear" {
          w785 = FALSE  # Mirror Second Leg?
          w786 = FALSE  # Mirror First Leg?
          n120 = Bundle By Name(cluster=w788, "First Path"="L1LeftToLRR" ("motionProfilePathName"), "Second Path Needed?"=FALSE, "Second Path"="BLANK") -> (w795:T2)
          n121 = Bundle By Name(cluster=w788, "First Path"="LRRToLeftLoadingStationA" ("motionProfilePathName"), "Second Path Needed?"=TRUE, "Second Path"="LRRToLeftLoadingStationB") -> (w787:T2)
        }
        frame "Right_Rocket_Rear" {
          w797 = TRUE  # Mirror Second Leg?
          w798 = TRUE  # Mirror First Leg?
          n122 = Bundle By Name(cluster=w800, "First Path"="L1LeftToLRR" ("motionProfilePathName"), "Second Path Needed?"=FALSE, "Second Path"="BLANK") -> (w807:T2)
          n123 = Bundle By Name(cluster=w800, "First Path"="LRRToLeftLoadingStationA" ("motionProfilePathName"), "Second Path Needed?"=TRUE, "Second Path"="LRRToLeftLoadingStationB") -> (w799:T2)
        }
      }
    }
    frame "Left L2" {
      n124 = case shown="\"5\"" w810 {
        tunnel: T2 {"First Path"="", "Second Path Needed?"=TRUE, "Second Path"=""} ("pathLeg") -> [w824 w831 w838 w845 w852 w859 w866 w873 w880 w887 w894 w901]
        tunnel: [w823 w830 w837 w844 w851 w858 w865 w872 w879 w886 w893 w900] -> w814
        tunnel: [w822 w829 w836 w843 w850 w857 w864 w871 w878 w885 w892 w899] -> w813
        tunnel: [TRUE ("Valid Path?") FALSE ("Valid Path?") TRUE ("Valid Path?") FALSE ("Valid Path?") TRUE ("Valid Path?") w856 TRUE ("Valid Path?") TRUE ("Valid Path?") TRUE ("Valid Path?") FALSE ("Valid Path?") TRUE ("Valid Path?") FALSE ("Valid Path?")] -> w808
        frame "1" {
          w822 = FALSE  # Mirror Third Leg?
          n125 = Bundle By Name(cluster=w824, "First Path"="LeftLoadingStationToCargo1" ("motionProfilePathName"), "Second Path Needed?"=FALSE, "Second Path"="BLANK") -> (w823:T2)
        }
        frame "2" {
          w829 = FALSE  # Mirror Third Leg?
          n126 = Bundle By Name(cluster=w831, "First Path"="LeftLoadingStationToCargo1" ("motionProfilePathName"), "Second Path Needed?"=FALSE, "Second Path"="BLANK") -> (w830:T2)
        }
        frame "3" {
          w836 = FALSE  # Mirror Third Leg?
          n127 = Bundle By Name(cluster=w838, "First Path"="LeftLoadingStationToCargo3" ("motionProfilePathName"), "Second Path Needed?"=FALSE, "Second Path"="BLANK") -> (w837:T2)
        }
        frame "4" {
          w843 = FALSE  # Mirror Third Leg?
          n128 = Bundle By Name(cluster=w845, "First Path"="LeftLoadingStationToCargo3" ("motionProfilePathName"), "Second Path Needed?"=FALSE, "Second Path"="BLANK") -> (w844:T2)
        }
        frame "5" {
          w850 = FALSE  # Mirror Third Leg?
          n129 = Bundle By Name(cluster=w852, "First Path"="LeftLoadingStationToCargo5" ("motionProfilePathName"), "Second Path Needed?"=FALSE, "Second Path"="BLANK") -> (w851:T2)
        }
        frame "6" {
          w856 = FALSE  # Valid Path?
          w857 = FALSE  # Mirror Third Leg?
          n130 = Bundle By Name(cluster=w859, "First Path"="LeftLoadingStationToCargo5" ("motionProfilePathName"), "Second Path Needed?"=FALSE, "Second Path"="BLANK") -> (w858:T2)
        }
        frame "7" {
          w864 = FALSE  # Mirror Third Leg?
          n131 = Bundle By Name(cluster=w866, "First Path"="LeftLoadingStationToCargo7" ("motionProfilePathName"), "Second Path Needed?"=FALSE, "Second Path"="BLANK") -> (w865:T2)
        }
        frame "8" {
          w871 = FALSE  # Mirror Third Leg?
          n132 = Bundle By Name(cluster=w873, "First Path"="LeftLoadingStationToCargo8" ("motionProfilePathName"), "Second Path Needed?"=FALSE, "Second Path"="BLANK") -> (w872:T2)
        }
        frame "Left_Rocket_Front" {
          w878 = FALSE  # Mirror Third Leg?
          n133 = Bundle By Name(cluster=w880, "First Path"="LeftLoadingStationToLRF" ("motionProfilePathName"), "Second Path Needed?"=FALSE, "Second Path"="BLANK") -> (w879:T2)
        }
        frame "Right_Rocket_Front" {
          w885 = FALSE  # Mirror Third Leg?
          n134 = Bundle By Name(cluster=w887, "First Path"="LeftLoadingStationToLRF" ("motionProfilePathName"), "Second Path Needed?"=FALSE, "Second Path"="BLANK") -> (w886:T2)
        }
        frame "Left_Rocket_Rear", Default {
          w892 = FALSE  # Mirror Third Leg?
          n135 = Bundle By Name(cluster=w894, "First Path"="LeftLoadingStationToLRR" ("motionProfilePathName"), "Second Path Needed?"=FALSE, "Second Path"="BLANK") -> (w893:T2)
        }
        frame "Right_Rocket_Rear" {
          w899 = FALSE  # Mirror Third Leg?
          n136 = Bundle By Name(cluster=w901, "First Path"="LeftLoadingStationToLRR" ("motionProfilePathName"), "Second Path Needed?"=FALSE, "Second Path"="BLANK") -> (w900:T2)
        }
      }
      n137 = case shown="\"7\", Default" w812 {
        tunnel: T2 {"First Path"="", "Second Path Needed?"=TRUE, "Second Path"=""} ("pathLeg") -> [w909 w921 w933 w945 w958 w970 w981 w993 w1005 w1017 w1029 w1041]
        tunnel: [w916 w928 w940 w952 w964 w976 w988 w1000 w1012 w1024 w1036 w1048] -> w819
        tunnel: [w908 w920 w932 w944 w957 w969 w980 w992 w1004 w1016 w1028 w1040] -> w816
        tunnel: [w907 w919 w931 w943 w956 w968 w979 w991 w1003 w1015 w1027 w1039] -> w818
        tunnel: [w906 w918 w930 w942 w955 w967 w978 w990 w1002 w1014 w1026 w1038] -> w817
        tunnel: w811 -> [_ _ _ _ _ _ _ _ _ _ _ _]
        tunnel: [FALSE ("Valid Path?") FALSE ("Valid Path?") FALSE ("Valid Path?") FALSE ("Valid Path?") FALSE ("Valid Path?") FALSE ("Valid Path?") TRUE ("Valid Path?") FALSE ("Valid Path?") w1001 FALSE ("Valid Path?") FALSE ("Valid Path?") FALSE ("Valid Path?")] -> w809
        frame "1" {
          w906 = FALSE  # Mirror Second Leg?
          w907 = FALSE  # Mirror First Leg?
          n138 = Bundle By Name(cluster=w909, "First Path"="L1LeftToCargo1" ("motionProfilePathName"), "Second Path Needed?"=FALSE, "Second Path"="BLANK") -> (w916:T2)
          n139 = Bundle By Name(cluster=w909, "First Path"="Cargo1ToLeftLoadingStation" ("motionProfilePathName"), "Second Path Needed?"=TRUE, "Second Path"="LRFToLeftLoadingStationB") -> (w908:T2)
        }
        frame "2" {
          w918 = FALSE  # Mirror Second Leg?
          w919 = FALSE  # Mirror First Leg?
          n140 = Bundle By Name(cluster=w921, "First Path"="L1LeftToCargo1" ("motionProfilePathName"), "Second Path Needed?"=FALSE, "Second Path"="BLANK") -> (w928:T2)
          n141 = Bundle By Name(cluster=w921, "First Path"="Cargo1ToLeftLoadingStation" ("motionProfilePathName"), "Second Path Needed?"=TRUE, "Second Path"="LRFToLeftLoadingStationB") -> (w920:T2)
        }
        frame "3" {
          w930 = FALSE  # Mirror Second Leg?
          w931 = FALSE  # Mirror First Leg?
          n142 = Bundle By Name(cluster=w933, "First Path"="L1LeftToCargo3" ("motionProfilePathName"), "Second Path Needed?"=FALSE, "Second Path"="BLANK") -> (w940:T2)
          n143 = Bundle By Name(cluster=w933, "First Path"="Cargo3ToLeftLoadingStation" ("motionProfilePathName"), "Second Path Needed?"=TRUE, "Second Path"="LRFToLeftLoadingStationB") -> (w932:T2)
        }
        frame "4" {
          w942 = FALSE  # Mirror Second Leg?
          w943 = FALSE  # Mirror First Leg?
          n144 = Bundle By Name(cluster=w945, "First Path"="L1LeftToCargo3" ("motionProfilePathName"), "Second Path Needed?"=FALSE, "Second Path"="BLANK") -> (w952:T2)
          n145 = Bundle By Name(cluster=w945, "First Path"="Cargo3ToLeftLoadingStation" ("motionProfilePathName"), "Second Path Needed?"=TRUE, "Second Path"="LRFToLeftLoadingStationB") -> (w944:T2)
        }
        frame "5" {
          w955 = FALSE  # Mirror Second Leg?
          w956 = FALSE  # Mirror First Leg?
          (unwired) "Cargo5ToLeftLoadingStationB" ("Second Path")
          n146 = Bundle By Name(cluster=w958, "First Path"="L1LeftToCargo5" ("motionProfilePathName"), "Second Path Needed?"=FALSE, "Second Path"="BLANK") -> (w964:T2)
          n147 = Bundle By Name(cluster=w958, "First Path"="Cargo5ToLeftLoadingStation" ("motionProfilePathName"), "Second Path Needed?"=TRUE, "Second Path"="BLANK") -> (w957:T2)
        }
        frame "6" {
          w967 = FALSE  # Mirror Second Leg?
          w968 = FALSE  # Mirror First Leg?
          (unwired) "Cargo5ToLeftLoadingStationB" ("Second Path")
          n148 = Bundle By Name(cluster=w970, "First Path"="L1LeftToCargo5" ("motionProfilePathName"), "Second Path Needed?"=FALSE, "Second Path"="BLANK") -> (w976:T2)
          n149 = Bundle By Name(cluster=w970, "First Path"="Cargo5ToLeftLoadingStation" ("motionProfilePathName"), "Second Path Needed?"=TRUE, "Second Path"="BLANK") -> (w969:T2)
        }
        frame "7", Default {
          w978 = FALSE  # Mirror Second Leg?
          w979 = FALSE  # Mirror First Leg?
          n150 = Bundle By Name(cluster=w981, "First Path"="low_L2LeftToCargo7" ("motionProfilePathName"), "Second Path Needed?"=FALSE, "Second Path"="BLANK") -> (w988:T2)
          n151 = Bundle By Name(cluster=w981, "First Path"="Cargo7ToLeftLoadingStationA" ("motionProfilePathName"), "Second Path Needed?"=TRUE, "Second Path"="Cargo7ToLeftLoadingStationB") -> (w980:T2)
        }
        frame "8" {
          w990 = FALSE  # Mirror Second Leg?
          w991 = FALSE  # Mirror First Leg?
          n152 = Bundle By Name(cluster=w993, "First Path"="L1LeftToCargo8" ("motionProfilePathName"), "Second Path Needed?"=FALSE, "Second Path"="BLANK") -> (w1000:T2)
          n153 = Bundle By Name(cluster=w993, "First Path"="Cargo8ToLeftLoadingStation" ("motionProfilePathName"), "Second Path Needed?"=TRUE, "Second Path"="Cargo7ToLeftLoadingStationB") -> (w992:T2)
        }
        frame "Left_Rocket_Front" {
          w1001 = FALSE  # Valid Path?
          w1002 = FALSE  # Mirror Second Leg?
          w1003 = FALSE  # Mirror First Leg?
          n154 = Bundle By Name(cluster=w1005, "First Path"="L1LeftToLRF" ("motionProfilePathName"), "Second Path Needed?"=FALSE, "Second Path"="BLANK") -> (w1012:T2)
          n155 = Bundle By Name(cluster=w1005, "First Path"="LRFToLeftLoadingStationA" ("motionProfilePathName"), "Second Path Needed?"=TRUE, "Second Path"="LRFToLeftLoadingStationB") -> (w1004:T2)
        }
        frame "Left_Rocket_Rear" {
          w1014 = FALSE  # Mirror Second Leg?
          w1015 = FALSE  # Mirror First Leg?
          n156 = Bundle By Name(cluster=w1017, "First Path"="L1LeftToLRR" ("motionProfilePathName"), "Second Path Needed?"=FALSE, "Second Path"="BLANK") -> (w1024:T2)
          n157 = Bundle By Name(cluster=w1017, "First Path"="LRRToLeftLoadingStationA" ("motionProfilePathName"), "Second Path Needed?"=TRUE, "Second Path"="LRRToLeftLoadingStationB") -> (w1016:T2)
        }
        frame "Right_Rocket_Rear" {
          w1026 = FALSE  # Mirror Second Leg?
          w1027 = FALSE  # Mirror First Leg?
          n158 = Bundle By Name(cluster=w1029, "First Path"="L1LeftToLRR" ("motionProfilePathName"), "Second Path Needed?"=FALSE, "Second Path"="BLANK") -> (w1036:T2)
          n159 = Bundle By Name(cluster=w1029, "First Path"="LRRToLeftLoadingStationA" ("motionProfilePathName"), "Second Path Needed?"=TRUE, "Second Path"="LRRToLeftLoadingStationB") -> (w1028:T2)
        }
        frame "Right_Rocket_Front" {
          w1038 = FALSE  # Mirror Second Leg?
          w1039 = FALSE  # Mirror First Leg?
          n160 = Bundle By Name(cluster=w1041, "First Path"="L1LeftToLRR" ("motionProfilePathName"), "Second Path Needed?"=FALSE, "Second Path"="BLANK") -> (w1048:T2)
          n161 = Bundle By Name(cluster=w1041, "First Path"="LRRToLeftLoadingStationA" ("motionProfilePathName"), "Second Path Needed?"=TRUE, "Second Path"="LRRToLeftLoadingStationB") -> (w1040:T2)
        }
      }
    }
    frame "Right L2" {
      n162 = case shown="\"8\"" w1053 {
        tunnel: T2 {"First Path"="", "Second Path Needed?"=TRUE, "Second Path"=""} ("pathLeg") -> [w1150 w1162 w1174 w1186 w1199 w1211 w1222 w1234 w1246 w1258 w1270 w1282]
        tunnel: [w1157 w1169 w1181 w1193 w1205 w1217 w1229 w1241 w1253 w1265 w1277 w1289] -> w1060
        tunnel: [w1149 w1161 w1173 w1185 w1198 w1210 w1221 w1233 w1245 w1257 w1269 w1281] -> w1057
        tunnel: [w1148 w1160 w1172 w1184 w1197 w1209 w1220 w1232 w1244 w1256 w1268 w1280] -> w1059
        tunnel: [w1147 w1159 w1171 w1183 w1196 w1208 w1219 w1231 w1243 w1255 w1267 w1279] -> w1058
        tunnel: w1052 -> [_ _ _ _ _ _ _ _ _ _ _ _]
        tunnel: [FALSE FALSE FALSE FALSE FALSE FALSE FALSE TRUE FALSE FALSE FALSE FALSE] -> w1050
        frame "1" {
          (unwired) TRUE  # Valid Path?
          w1147 = FALSE  # Mirror Second Leg?
          w1148 = FALSE  # Mirror First Leg?
          n163 = Bundle By Name(cluster=w1150, "First Path"="L1LeftToCargo1" ("motionProfilePathName"), "Second Path Needed?"=FALSE, "Second Path"="BLANK") -> (w1157:T2)
          n164 = Bundle By Name(cluster=w1150, "First Path"="Cargo1ToLeftLoadingStation" ("motionProfilePathName"), "Second Path Needed?"=TRUE, "Second Path"="LRFToLeftLoadingStationB") -> (w1149:T2)
        }
        frame "2" {
          w1159 = TRUE  # Mirror Second Leg?
          w1160 = TRUE  # Mirror First Leg?
          n165 = Bundle By Name(cluster=w1162, "First Path"="L1LeftToCargo1" ("motionProfilePathName"), "Second Path Needed?"=FALSE, "Second Path"="BLANK") -> (w1169:T2)
          n166 = Bundle By Name(cluster=w1162, "First Path"="Cargo1ToLeftLoadingStation" ("motionProfilePathName"), "Second Path Needed?"=TRUE, "Second Path"="LRFToLeftLoadingStationB") -> (w1161:T2)
        }
        frame "3" {
          w1171 = FALSE  # Mirror Second Leg?
          w1172 = FALSE  # Mirror First Leg?
          n167 = Bundle By Name(cluster=w1174, "First Path"="L1LeftToCargo3" ("motionProfilePathName"), "Second Path Needed?"=FALSE, "Second Path"="BLANK") -> (w1181:T2)
          n168 = Bundle By Name(cluster=w1174, "First Path"="Cargo3ToLeftLoadingStation" ("motionProfilePathName"), "Second Path Needed?"=TRUE, "Second Path"="LRFToLeftLoadingStationB") -> (w1173:T2)
        }
        frame "4" {
          w1183 = TRUE  # Mirror Second Leg?
          w1184 = TRUE  # Mirror First Leg?
          n169 = Bundle By Name(cluster=w1186, "First Path"="L1LeftToCargo3" ("motionProfilePathName"), "Second Path Needed?"=FALSE, "Second Path"="BLANK") -> (w1193:T2)
          n170 = Bundle By Name(cluster=w1186, "First Path"="Cargo3ToLeftLoadingStation" ("motionProfilePathName"), "Second Path Needed?"=TRUE, "Second Path"="LRFToLeftLoadingStationB") -> (w1185:T2)
        }
        frame "5" {
          w1196 = FALSE  # Mirror Second Leg?
          w1197 = FALSE  # Mirror First Leg?
          (unwired) "Cargo5ToLeftLoadingStationB" ("Second Path")
          n171 = Bundle By Name(cluster=w1199, "First Path"="L1LeftToCargo5" ("motionProfilePathName"), "Second Path Needed?"=FALSE, "Second Path"="BLANK") -> (w1205:T2)
          n172 = Bundle By Name(cluster=w1199, "First Path"="Cargo5ToLeftLoadingStation" ("motionProfilePathName"), "Second Path Needed?"=TRUE, "Second Path"="BLANK") -> (w1198:T2)
        }
        frame "6" {
          w1208 = TRUE  # Mirror Second Leg?
          w1209 = TRUE  # Mirror First Leg?
          (unwired) "Cargo5ToLeftLoadingStationB" ("Second Path")
          n173 = Bundle By Name(cluster=w1211, "First Path"="L1LeftToCargo5" ("motionProfilePathName"), "Second Path Needed?"=FALSE, "Second Path"="BLANK") -> (w1217:T2)
          n174 = Bundle By Name(cluster=w1211, "First Path"="Cargo5ToLeftLoadingStation" ("motionProfilePathName"), "Second Path Needed?"=TRUE, "Second Path"="BLANK") -> (w1210:T2)
        }
        frame "7", Default {
          w1219 = FALSE  # Mirror Second Leg?
          w1220 = FALSE  # Mirror First Leg?
          n175 = Bundle By Name(cluster=w1222, "First Path"="L1LeftToCargo7" ("motionProfilePathName"), "Second Path Needed?"=FALSE, "Second Path"="BLANK") -> (w1229:T2)
          n176 = Bundle By Name(cluster=w1222, "First Path"="Cargo7ToLeftLoadingStationA" ("motionProfilePathName"), "Second Path Needed?"=TRUE, "Second Path"="Cargo7ToLeftLoadingStationB") -> (w1221:T2)
        }
        frame "8" {
          w1231 = FALSE  # Mirror Second Leg?
          w1232 = FALSE  # Mirror First Leg?
          n177 = Bundle By Name(cluster=w1234, "First Path"="low_L2RightToCargo8" ("motionProfilePathName"), "Second Path Needed?"=FALSE, "Second Path"="BLANK") -> (w1241:T2)
          n178 = Bundle By Name(cluster=w1234, "First Path"="Cargo8ToRightLoadingStationA" ("motionProfilePathName"), "Second Path Needed?"=TRUE, "Second Path"="low_Cargo8ToRightLoadingStationA") -> (w1233:T2)
        }
        frame "Left_Rocket_Front" {
          w1243 = FALSE  # Mirror Second Leg?
          w1244 = FALSE  # Mirror First Leg?
          n179 = Bundle By Name(cluster=w1246, "First Path"="L1LeftToLRF" ("motionProfilePathName"), "Second Path Needed?"=FALSE, "Second Path"="BLANK") -> (w1253:T2)
          n180 = Bundle By Name(cluster=w1246, "First Path"="LRFToLeftLoadingStationA" ("motionProfilePathName"), "Second Path Needed?"=TRUE, "Second Path"="LRFToLeftLoadingStationB") -> (w1245:T2)
        }
        frame "Left_Rocket_Rear" {
          w1255 = FALSE  # Mirror Second Leg?
          w1256 = FALSE  # Mirror First Leg?
          n181 = Bundle By Name(cluster=w1258, "First Path"="L1LeftToLRR" ("motionProfilePathName"), "Second Path Needed?"=FALSE, "Second Path"="BLANK") -> (w1265:T2)
          n182 = Bundle By Name(cluster=w1258, "First Path"="LRRToLeftLoadingStationA" ("motionProfilePathName"), "Second Path Needed?"=TRUE, "Second Path"="LRRToLeftLoadingStationB") -> (w1257:T2)
        }
        frame "Right_Rocket_Rear" {
          w1267 = TRUE  # Mirror Second Leg?
          w1268 = TRUE  # Mirror First Leg?
          n183 = Bundle By Name(cluster=w1270, "First Path"="L1LeftToLRR" ("motionProfilePathName"), "Second Path Needed?"=FALSE, "Second Path"="BLANK") -> (w1277:T2)
          n184 = Bundle By Name(cluster=w1270, "First Path"="LRRToLeftLoadingStationA" ("motionProfilePathName"), "Second Path Needed?"=TRUE, "Second Path"="LRRToLeftLoadingStationB") -> (w1269:T2)
        }
        frame "Right_Rocket_Front" {
          w1279 = TRUE  # Mirror Second Leg?
          w1280 = TRUE  # Mirror First Leg?
          n185 = Bundle By Name(cluster=w1282, "First Path"="L1LeftToLRR" ("motionProfilePathName"), "Second Path Needed?"=FALSE, "Second Path"="BLANK") -> (w1289:T2)
          n186 = Bundle By Name(cluster=w1282, "First Path"="LRRToLeftLoadingStationA" ("motionProfilePathName"), "Second Path Needed?"=TRUE, "Second Path"="LRRToLeftLoadingStationB") -> (w1281:T2)
        }
      }
      n187 = case shown="\"6\"" w1051 {
        tunnel: T2 {"First Path"="", "Second Path Needed?"=TRUE, "Second Path"=""} ("pathLeg") -> [w1065 w1072 w1079 w1086 w1093 w1100 w1107 w1114 w1121 w1128 w1135 w1142]
        tunnel: [w1064 w1071 w1078 w1085 w1092 w1099 w1106 w1113 w1120 w1127 w1134 w1141] -> w1055
        tunnel: [w1063 w1070 w1077 w1084 w1091 w1098 w1105 w1112 w1119 w1126 w1133 w1140] -> w1054
        tunnel: [FALSE TRUE FALSE TRUE FALSE TRUE TRUE TRUE FALSE TRUE FALSE TRUE] -> w1049
        frame "1" {
          w1063 = FALSE  # Mirror Third Leg?
          n188 = Bundle By Name(cluster=w1065, "First Path"="LeftLoadingStationToCargo1" ("motionProfilePathName"), "Second Path Needed?"=FALSE, "Second Path"="BLANK") -> (w1064:T2)
        }
        frame "2" {
          w1070 = TRUE  # Mirror Third Leg?
          n189 = Bundle By Name(cluster=w1072, "First Path"="LeftLoadingStationToCargo1" ("motionProfilePathName"), "Second Path Needed?"=FALSE, "Second Path"="BLANK") -> (w1071:T2)
        }
        frame "3" {
          w1077 = FALSE  # Mirror Third Leg?
          n190 = Bundle By Name(cluster=w1079, "First Path"="LeftLoadingStationToCargo3" ("motionProfilePathName"), "Second Path Needed?"=FALSE, "Second Path"="BLANK") -> (w1078:T2)
        }
        frame "4" {
          w1084 = TRUE  # Mirror Third Leg?
          n191 = Bundle By Name(cluster=w1086, "First Path"="LeftLoadingStationToCargo3" ("motionProfilePathName"), "Second Path Needed?"=FALSE, "Second Path"="BLANK") -> (w1085:T2)
        }
        frame "5" {
          w1091 = FALSE  # Mirror Third Leg?
          n192 = Bundle By Name(cluster=w1093, "First Path"="LeftLoadingStationToCargo5" ("motionProfilePathName"), "Second Path Needed?"=FALSE, "Second Path"="BLANK") -> (w1092:T2)
        }
        frame "6" {
          w1098 = TRUE  # Mirror Third Leg?
          n193 = Bundle By Name(cluster=w1100, "First Path"="LeftLoadingStationToCargo5" ("motionProfilePathName"), "Second Path Needed?"=FALSE, "Second Path"="BLANK") -> (w1099:T2)
        }
        frame "7" {
          w1105 = TRUE  # Mirror Third Leg?
          n194 = Bundle By Name(cluster=w1107, "First Path"="LeftLoadingStationToCargo8" ("motionProfilePathName"), "Second Path Needed?"=FALSE, "Second Path"="BLANK") -> (w1106:T2)
        }
        frame "8" {
          w1112 = TRUE  # Mirror Third Leg?
          n195 = Bundle By Name(cluster=w1114, "First Path"="LeftLoadingStationToCargo7" ("motionProfilePathName"), "Second Path Needed?"=FALSE, "Second Path"="BLANK") -> (w1113:T2)
        }
        frame "Left_Rocket_Front" {
          w1119 = FALSE  # Mirror Third Leg?
          n196 = Bundle By Name(cluster=w1121, "First Path"="LeftLoadingStationToLRF" ("motionProfilePathName"), "Second Path Needed?"=FALSE, "Second Path"="BLANK") -> (w1120:T2)
        }
        frame "Right_Rocket_Front" {
          w1126 = TRUE  # Mirror Third Leg?
          n197 = Bundle By Name(cluster=w1128, "First Path"="LeftLoadingStationToLRF" ("motionProfilePathName"), "Second Path Needed?"=FALSE, "Second Path"="BLANK") -> (w1127:T2)
        }
        frame "Left_Rocket_Rear", Default {
          w1133 = FALSE  # Mirror Third Leg?
          n198 = Bundle By Name(cluster=w1135, "First Path"="LeftLoadingStationToLRR" ("motionProfilePathName"), "Second Path Needed?"=FALSE, "Second Path"="BLANK") -> (w1134:T2)
        }
        frame "Right_Rocket_Rear" {
          w1140 = TRUE  # Mirror Third Leg?
          n199 = Bundle By Name(cluster=w1142, "First Path"="LeftLoadingStationToLRR" ("motionProfilePathName"), "Second Path Needed?"=FALSE, "Second Path"="BLANK") -> (w1141:T2)
        }
      }
    }
  }
  n200 = Unbundle By Name(w42) -> ("Second Path"=w35:string)
  n201 = Unbundle By Name(w42) -> ("First Path"=w38:string)
  n202 = Unbundle By Name(w46) -> ("Second Path"=w15:string)
  n203 = Unbundle By Name(w43) -> ("Second Path"=w23:string)
  n204 = And(x=w8, y=w7) -> (x .and. y?=→"Complete Path Valid?":bool)
  n205 = Unbundle By Name(w46) -> ("First Path"=w18:string)
  n206 = Unbundle By Name(w43) -> ("First Path"=w20:string)
  n207 = Concatenate Strings(w38, "_MIR" ("string")) -> (w34:string)
  n208 = Concatenate Strings(w35, "_MIR" ("string")) -> (w33:string)
  n209 = Not(x=w41) -> (.not. x?=w30:bool)
  n210 = Concatenate Strings(w18, "_MIR" ("string")) -> (w14:string)
  n211 = Concatenate Strings(w15, "_MIR" ("string")) -> (w13:string)
  n212 = Concatenate Strings(w20, "_MIR" ("string")) -> (w24:string)
  n213 = Concatenate Strings(w23, "_MIR" ("string")) -> (w25:string)
  n214 = Bundle By Name(cluster=w42, "First Path"=w34) -> (w32:T2)
  n215 = Bundle By Name(cluster=w32, "Second Path"=w33) -> (w31:T2)
  n216 = Not(x=w45) -> (.not. x?=w9:bool)
  n217 = Not(x=w44) -> (.not. x?=w28:bool)
  n218 = Bundle By Name(cluster=w46, "First Path"=w14) -> (w12:T2)
  n219 = Bundle By Name(cluster=w12, "Second Path"=w13) -> (w11:T2)
  n220 = Bundle By Name(cluster=w43, "First Path"=w24) -> (w26:T2)
  n221 = Bundle By Name(cluster=w26, "Second Path"=w25) -> (w27:T2)
  n222 = Select(t=w42, s=w30, f=w31) -> (s? t:f=→"Score Second HP Leg":T2)
  n223 = Select(t=w46, s=w9, f=w11) -> (s? t:f=→"Score First HP Leg":T2)
  n224 = Select(t=w43, s=w28, f=w27) -> (s? t:f=→"Retrieve Second HP Leg":T2)
